vi "dfd_Convert SOS Coefficients to String.vi"(5 "indent order":i32, 7 "format string":string="%-+024.16e", 11 "filter coef":T1) -> (2 "gain":dbl, 3 "XML string out":string)   [LabVIEW 2017, in "NI_DigFilter_Process.lvlib"]
uses:
  <vilib>/addons/Digital Filter Design/NI_DigFilter_Process.lvlib
  <vilib>/addons/Digital Filter Design/_Objects.llb/DFD Filter Coef.ctl
  <vilib>/addons/Digital Filter Design/_Objects.llb/DFD Filter Structure Type Selector.ctl
  <vilib>/addons/Digital Filter Design/NI_DigFilterLicensed.lvlib
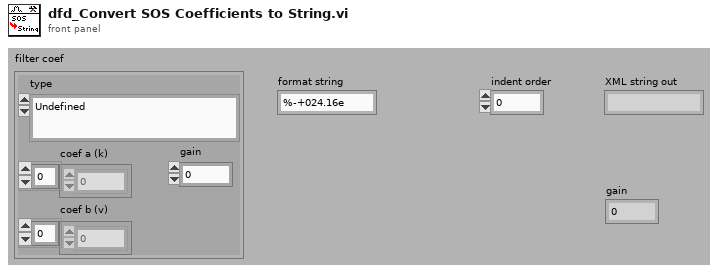
[diagram p1: front panel]
types:
  T1 = typedef "NI_DigFilterLicensed.lvlib/DFD Filter Coef.ctl" = cluster{"type":T2, "gain":dbl, "coef a (k)":dbl[], "coef b (v)":dbl[]}
  T2 = typedef "NI_DigFilterLicensed.lvlib/DFD Filter Structure Type Selector.ctl" = enum16{"Undefined", "FIR Direct Form", "FIR Direct Form Transposed", "FIR Symmetric", "FIR Antisymmetric", "IIR Direct Form I", "IIR Direct Form I Transposed", "IIR Direct Form II", "IIR Direct Form II Transposed", "IIR Cascaded Second Order Sections Form I", "IIR Cascaded Second Order Sections Form I Transposed", "IIR Cascaded Second Order Sections Form II", "IIR Cascaded Second Order Sections Form II Transposed", "Lattice Allpass (basic sections)", "Lattice Allpass (one multiplier sections)", "Lattice Allpass (normalized sections)", "Lattice AR (basic sections)", "Lattice AR (one multiplier sections)", "Lattice AR (normalized sections)", "Lattice MA (minimum phase)", "Lattice MA (maximum phase)", "Lattice ARMA (basic sections)", "Lattice ARMA (one multiplier sections)", "Lattice ARMA (normalized sections)"}
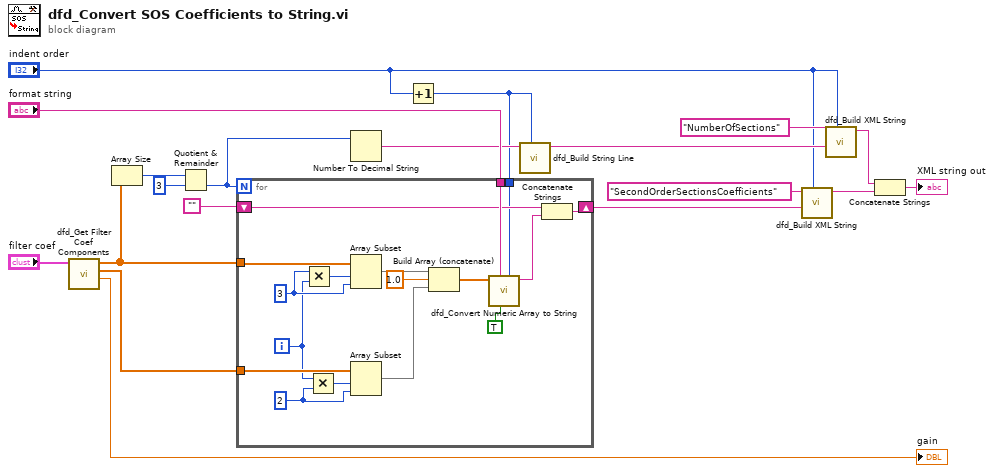
[diagram p0: block diagram]
diagram:
  n1 = call <vilib>:"dfd_Get Filter Coef Components.vi"("filter coef"="filter coef") -> ("gain"=→"gain":dbl, "coef a (k)"=w16:dbl[], "coef b (v)"=w17:dbl[])  [unwired: 1 in, 7 out]
  n2 = Array Size(array=w17) -> (size(s)=w19:i32)
  n3 = Quotient & Remainder(x=w19, y=3) -> (floor(x/y)=w3:i32)  [unwired: 1 out]
  n4 = Number To Decimal String(number=w3) -> (decimal integer string=w5:string)  [unwired: 1 out]
  n5 = Increment(x="indent order") -> (x+1=w4:i32)
  n6 = for {
    N: w3 -> [_]
    tunnel: w16 -> [w36]
    tunnel: w17 -> [w33]
    shift-right: [w20] -> w9
    shift-left: "" -> [w29]
    tunnel: w4 -> [w22]
    tunnel: "format string" -> [w31]
    i -> [w27]
    w32 = 3 ("y")
    w28 = 2 ("y")
    n7 = Multiply(x=w32, y=w27) -> (x*y=w34:i32)
    n8 = Multiply(x=w27, y=w28) -> (x*y=w35:i32)
    n9 = Array Subset(array=w33, index=w34, length=w32) -> (w26:dbl[])
    n10 = Array Subset(array=w36, index=w35, length=w28) -> (w24:dbl[])
    n11 = Build Array (concatenate)(w26, 1.0, w24) -> (w23:dbl[])
    n12 = call <vilib>:"dfd_Convert Numeric Array to String.vi"("indent order"=w22, "display in one line?"=TRUE, "format string"=w31, "numeric array"=w23) -> ("string"=w30:string)  [unwired: 2 in, 5 out]
    n13 = Concatenate Strings(w29, w30) -> (w20:string)
  }
  n14 = call <vilib>:"dfd_Build String Line.vi"("indent order"=w4, "string"=w5) -> ("string line"=w6:string)  [unwired: 9 out]
  n15 = call <vilib>:"dfd_Build XML String.vi"("indent order"="indent order", "string in"=w9, "element name"="SecondOrderSectionsCoefficients") -> ("xml string out"=w11:string)  [unwired: 1 in, 7 out]
  n16 = call <vilib>:"dfd_Build XML String.vi"("indent order"="indent order", "string in"=w6, "element name"="NumberOfSections") -> ("xml string out"=w8:string)  [unwired: 1 in, 7 out]
  n17 = Concatenate Strings(w8, w11) -> (→"XML string out":string)
